vi "sub_save_string_as_JSON_file.vi"(8 "error in (no error)":errorcluster, 10 "Value":string, 11 "appended path":path) -> (0 "error out":errorcluster)   [LabVIEW 2013, in "daqio minimal.lvlib"]
uses:
  daqio minimal.lvlib
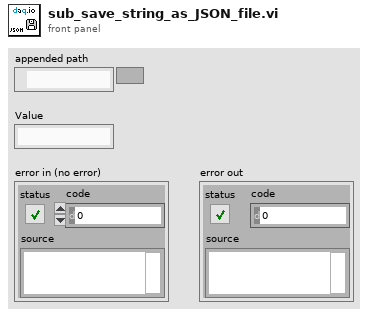
[diagram p1: front panel]
types:
  T1 = enum16{"open", "replace", "create", "open or create", "replace or create", "replace or create with confirmation"}
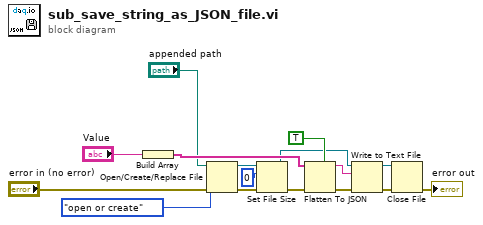
[diagram p0: block diagram]
diagram:
  n1 = Build Array("Value") -> (w16:string[])
  n2 = Open/Create/Replace File(file path (use dialog)="appended path", error in="error in (no error)", operation (0:open)=T1."open or create") -> (refnum out=w5:refnum<file>, error out=w3:errorcluster)  [unwired: 3 in, 1 out]
  n3 = Set File Size(4:w3, 6:i64 0 ("size (in bytes)"), 7:w5) -> (0:w6:errorcluster, 3:w8:refnum<file>)
  n4 = Flatten To JSON(enable LabVIEW extensions? (T)=TRUE, anything=w16, error in (no error)=w6) -> (JSON string=w7:string, 11:w9:errorcluster)
  n5 = Write to Text File(file (use dialog)=w8, text=w7, error in=w9) -> (refnum out=w11:refnum<file>, error out=w10:errorcluster)  [unwired: 1 in, 1 out]
  n6 = Close File(refnum=w11, error in=w10) -> (error out=→"error out":errorcluster)  [unwired: 1 out]
